vi "Power Scan batch.vi"(6 "File Path Control":path, 7 "Array - Numeric":dbl[][](array[numeric]), 8 "Z Position":dbl, 9 "RS232 settings":cluster{"Portnumber":i32, "Baudrate":u16}={"Portnumber"=12, "Baudrate"=5} {"Portnumber" items=["COM1", "COM2", "COM3", "COM4", "COM5", "COM6", "COM7", "COM8", "COM9", "COM10", "COM11", "COM12", "COM13", "COM14", "COM15", "COM16", "COM17", "COM18", "COM19", "COM20", "COM21", "COM22", "COM23", "COM24", "COM25", "COM26", "COM27", "COM28", "COM29", "COM30"]; "Baudrate" items=["9600", "14400", "19200", "38400", "57600", "115200"]}, 10 "Y Parameters":T1={"Number of Y Steps"=200, "Max Y (V)"=2.0, "Min Y (V)"=-2.0}, 11 "X Parameters":T2={"Number of X Steps"=200, "Max X (V)"=2.0, "Min X (V)"=-2.0}) -> (0 "Z Position 2":dbl)   [LabVIEW 2012]
uses:
  SPCM files/Global FIFO variabls.vi
panel:
  in  "Min (mW)":dbl
  in  "Max (mW)":dbl
  in  "# Steps":dbl
  out "Numeric":i32
  in  "stop":bool
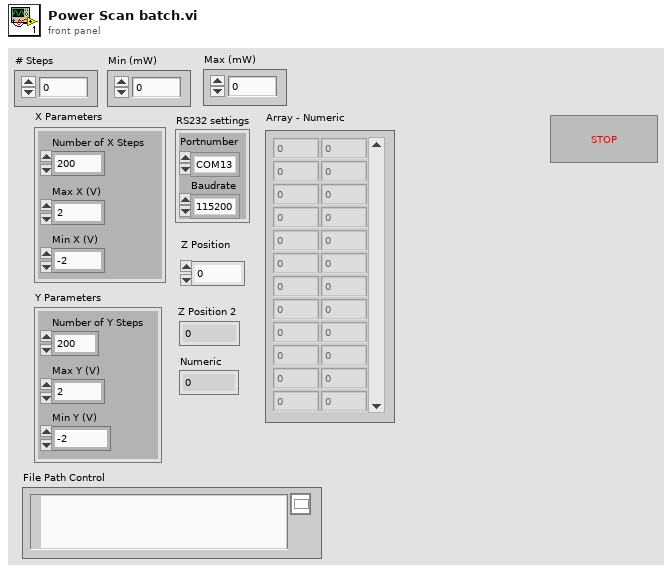
[diagram p1: front panel]
types:
  T1 = cluster{"Number of Y Steps":i32, "Max Y (V)":dbl, "Min Y (V)":dbl}
  T2 = cluster{"Number of X Steps":i32, "Max X (V)":dbl, "Min X (V)":dbl}
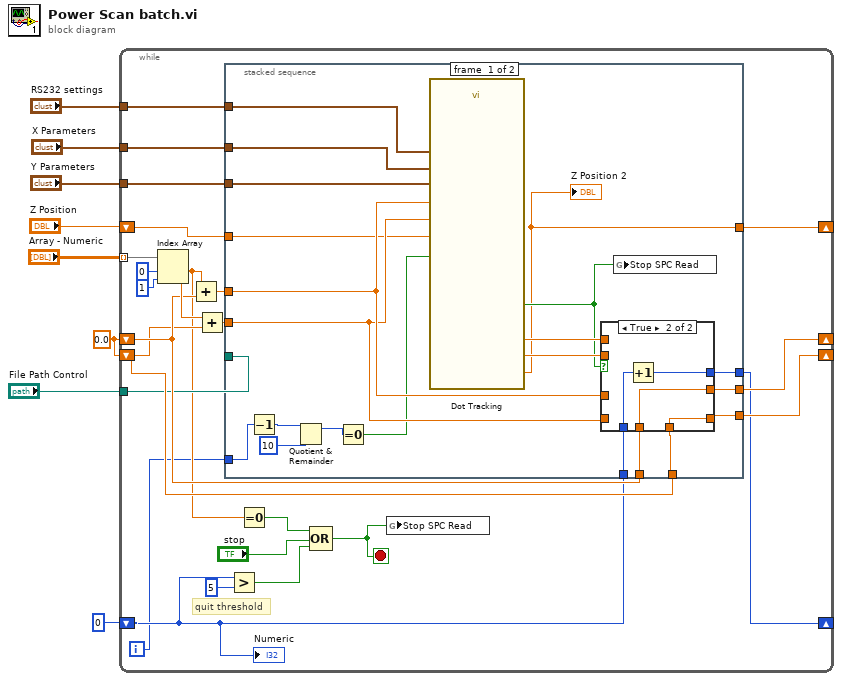
[diagram p0: block diagram]
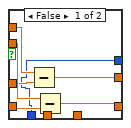
[diagram p2: hidden frame]
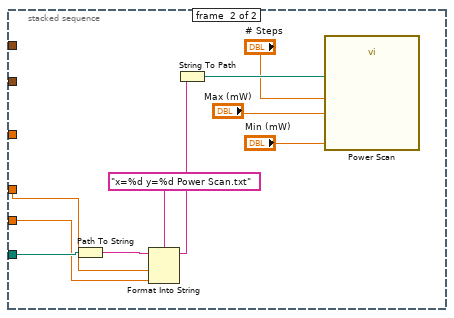
[diagram p3: hidden frame]
diagram:
  w4 = 0.0
  n1 = while {
    tunnel: "RS232 settings" -> [w33]
    tunnel: "X Parameters" -> [w32]
    tunnel: "Y Parameters" -> [w31]
    tunnel: "Array - Numeric" -> [w30] mode=indexing
    shift-right: [w24] -> _
    shift-left: w4 -> [w21]
    shift-right: [w23] -> _
    shift-left: w4 -> [w20]
    tunnel: "File Path Control" -> [w19]
    shift-right: [w14] -> _
    shift-left: "Z Position" -> [w22]
    shift-right: [w13] -> _
    shift-left: 0 -> [w12]
    i -> [w9]
    stop <- w15 stop-if-true
    # "quit threshold"
    n2 = Index Array(array=w30, index #1=0 ("index (row)"), index #2=1 ("index (row)")) -> (element #1=w18:dbl, element #2=w26:dbl)
    n3 = Add(x=w18, y=w21) -> (x+y=w27:dbl)
    n4 = Add(x=w26, y=w20) -> (x+y=w25:dbl)
    n5 = stacked-sequence {
      tunnel: w33 -> [w54 _]
      tunnel: w32 -> [w53 _]
      tunnel: w31 -> [w52 _]
      tunnel: w27 -> [w49 w72]
      tunnel: w25 -> [w48 w71]
      tunnel: [w47 _] -> w24
      tunnel: [w46 _] -> w23
      tunnel: w22 -> [w45 _]
      tunnel: w21 -> [w44 _]
      tunnel: w20 -> [w43 _]
      tunnel: w19 -> [_ w75]
      tunnel: [w41 _] -> w14
      tunnel: w12 -> [w40 _]
      tunnel: [w39 _] -> w13
      tunnel: w9 -> [w38 _]
      frame #0 {
        n6 = Decrement(x=w38) -> (x-1=w37:i32)
        n7 = Quotient & Remainder(x=w37, y=10) -> (x-y*floor(x/y)=w35:i32)  [unwired: 1 out]
        n8 = Equal To 0?(x=w35) -> (x = 0?=w34:bool)
        n9 = call "Dot Tracking.vi"("X"=w53, "Y Parameters"=w52, "RS232 settings"=w54, "X Pos"=w49, "Y pos"=w48, "Z Pos"=w45, "Z-track?"=w34) -> ("X Position"=w51:dbl, "Y Position"=w50:dbl, "Z Position"=w41:dbl, "Gave up?"=w42:bool)  [unwired: 2 in, 3 out]
        "Z Position 2" <- w41
        n10 = case shown="True" w42 {
          tunnel: w51 -> [w61 _]
          tunnel: w50 -> [w60 _]
          tunnel: w49 -> [w59 _]
          tunnel: w48 -> [w58 _]
          tunnel: [w57 w65] -> w47
          tunnel: [w56 w64] -> w46
          tunnel: w44 -> [_ w65]
          tunnel: w43 -> [_ w64]
          tunnel: w40 -> [w55 w63]
          tunnel: [w55 w62] -> w39
          frame False {
            n11 = Subtract(x=w61, y=w59) -> (x-y=w57:dbl)
            n12 = Subtract(x=w60, y=w58) -> (x-y=w56:dbl)
          }
          frame True {
            n13 = Increment(x=w63) -> (x+1=w62:i32)
          }
        }
        n14 = global write "Global FIFO variabls.vi" "Stop SPC Read"(w42) -> ()
      }
      frame #1 {
        n15 = Path To String(path=w75) -> (string=w73:string)
        n16 = Format Into String(format string="x=%d y=%d Power Scan.txt", initial string=w73, w72, w71) -> (resulting string=w70:string)  [unwired: 1 in, 1 out]
        n17 = String To Path(string=w70) -> (path=w69:path)
        n18 = call "Power Scan.vi"("# Steps"="# Steps", "Max (mW)"="Max (mW)", "Min (mW)"="Min (mW)", "file path (dialog if empty)"=w69) -> ()  [unwired: 7 in, 1 out]
      }
    }
    n19 = Greater?(x=w12, y=5) -> (0:w10:bool)
    n20 = Equal To 0?(x=w18) -> (x = 0?=w17:bool)
    n21 = Compound Arithmetic op=OR(w17, "stop", w10) -> (w15:bool)
    n22 = global write "Global FIFO variabls.vi" "Stop SPC Read"(w15) -> ()
    "Numeric" <- w12
  }
